vi "Compression with DCT.vi"() -> ()   [LabVIEW 2023]
doc: "This VI uses the DCT VI to compress images. LabVIEW transforms the Source Image to DCT Coefficients in 8-by-8 blocks, then the inverse DCT transforms the image back to Restored Image."
uses:
  Images/_Images.ctl
  <vilib>/Analysis/2dsp.llb/2D DCT.vi
  <vilib>/Analysis/2dsp.llb/2D Inverse DCT.vi
  <vilib>/Analysis/NI_AALPro.lvlib
panel:
  in  "Image Selector":T1=enum."Part1"
  out "DCT":T2(plugin-control)
  in  "Compression Level (1-max, 15 - min)":i32(slide)=4 scale=1.0..15.0
  out "min value":dbl
  out "max value":dbl
  out "Difference":T2(plugin-control)
  out "MSE":dbl
  out "PSNR (dB)":dbl
  out "Reconstructed Image":T2(plugin-control)
  out "Image":T2(plugin-control)
  out "Number of block size":i32
  out "Truncated Pattern":bool[][](array[boolean])=[[TRUE, TRUE, TRUE, TRUE, FALSE, FALSE, FALSE, FALSE], [TRUE, TRUE, TRUE, FALSE, FALSE, FALSE, FALSE, FALSE], [TRUE, TRUE, FALSE, FALSE, FALSE, FALSE, FALSE, FALSE], [TRUE, FALSE, FALSE, FALSE, FALSE, FALSE, FALSE, FALSE], [FALSE, FALSE, FALSE, FALSE, FALSE, FALSE, FALSE, FALSE], [FALSE, FALSE, FALSE, FALSE, FALSE, FALSE, FALSE, FALSE], [FALSE, FALSE, FALSE, FALSE, FALSE, FALSE, FALSE, FALSE], [FALSE, FALSE, FALSE, FALSE, FALSE, FALSE, FALSE, FALSE]]
  # "Image Compression and the Discrete Cosine Transform"
  # "Inverse DCT"
  # "DCT\n(8 X 8 block)"
  # "Modify the Truncated Pattern  and verify \nthat the Mean Square Error (MSE) \nreduces as you enable more bits."
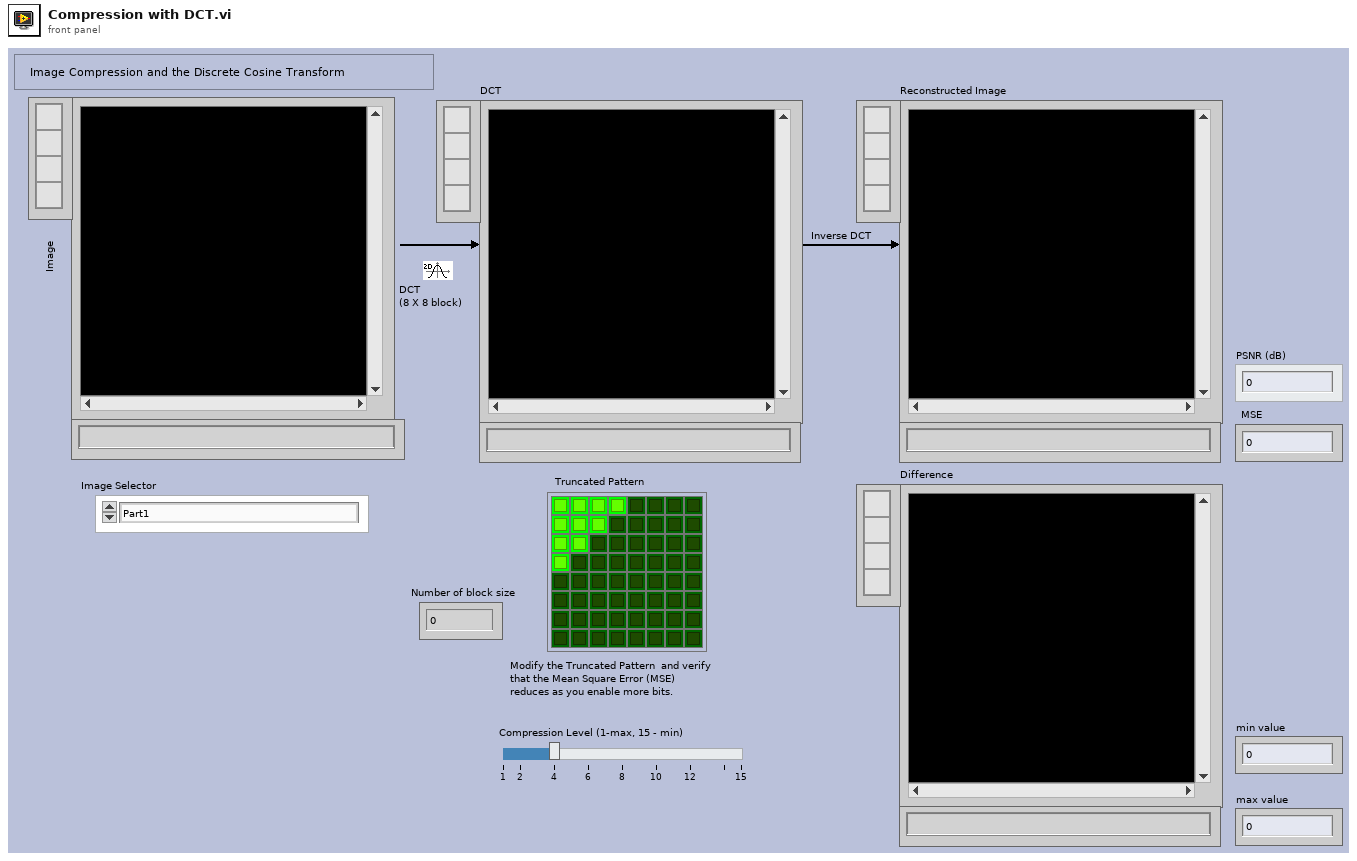
[diagram p1: front panel]
types:
  T1 = typedef "_Images.ctl" = enum16{"Balls2", "Battery1", "Battery2", "Connector1", "Subwoofer1", "Subwoofer2", "Subwoofer3", "Subwoofer4", "Hase1", "Lamp1", "Lamp2", "Mouse1", "PhotoLens1", "Po1", "PowerSupply1", "Router", "--- Step Wedges ---", "Stepwedge1", "Stepwedge2", "Stepwedge3", "--- Fusion ---", "Fusion160kV", "Fusion2-120kV", "Fusion2-320kV", "Fusion300kV", "FusionPart1-120kV", "FusionPart1-180kV", "--- PART 01 ---", "Part1", "Part2", "Part3", "Part4", "Part5", "Part6", "Part7", "Part8", "--- Different Integrations ---", "Step2737-02Int", "Step2737-04Int", "Step2737-08Int", "Step2737-16Int", "Step2737-32Int", "Step2737-64Int"}
  T2 = typedef "IMAQ Image.ctl" = refnum<image>
  T3 = typedef "Image Type" = u32
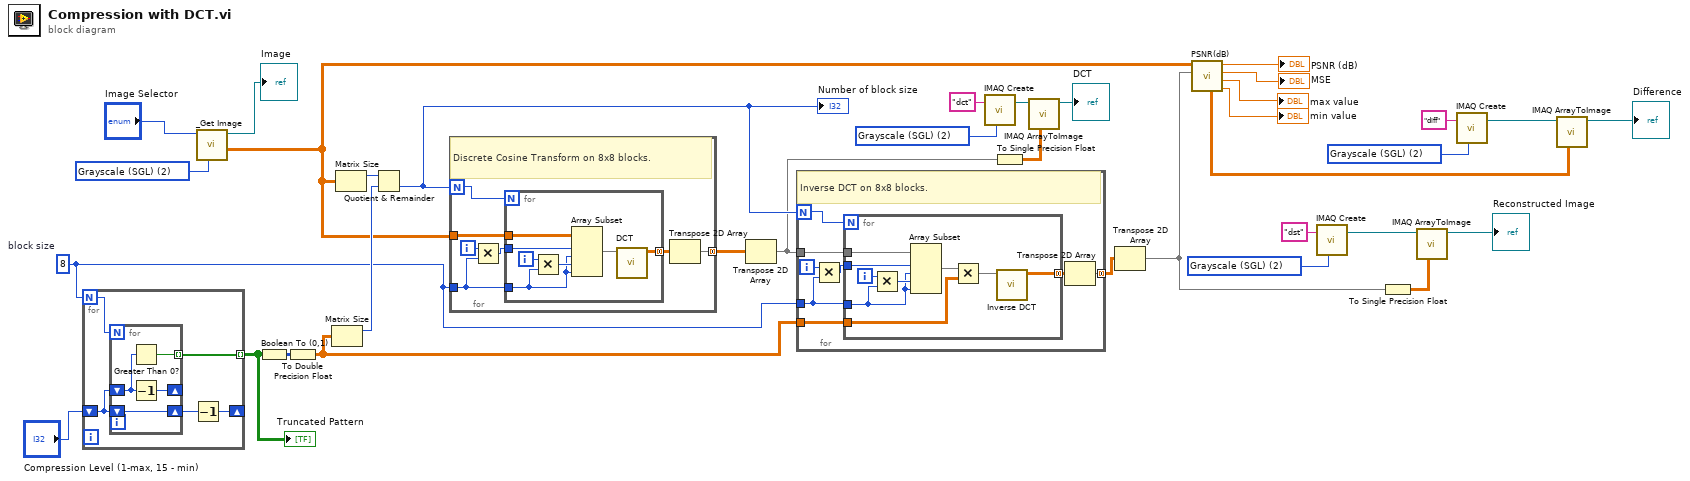
[diagram p0: block diagram]
diagram:
  w11 = T3 2 items=["Grayscale (U8)", "Grayscale (I16)", "Grayscale (SGL)", "Complex (CSG)", "RGB (U32)", "HSL (U32)", "RGB (U64)", "Grayscale (U16)"] ("Image Type")
  w19 = T3 2 items=["Grayscale (U8)", "Grayscale (I16)", "Grayscale (SGL)", "Complex (CSG)", "RGB (U32)", "HSL (U32)", "RGB (U64)", "Grayscale (U16)"] ("Image Type")
  w24 = T3 2 items=["Grayscale (U8)", "Grayscale (I16)", "Grayscale (SGL)", "Complex (CSG)", "RGB (U32)", "HSL (U32)", "RGB (U64)", "Grayscale (U16)"] ("Image Type (U16)")
  w26 = T3 2 items=["Grayscale (U8)", "Grayscale (I16)", "Grayscale (SGL)", "Complex (CSG)", "RGB (U32)", "HSL (U32)", "RGB (U64)", "Grayscale (U16)"] ("Image Type")
  w5 = 8  # block size
  n1 = for {
    N: w5 -> [w40]
    shift-right: [w37] -> _
    shift-left: "Compression Level (1-max, 15 - min)" -> [w38]
    tunnel: [w36] -> w14 mode=indexing
    n2 = for {
      N: w40 -> [_]
      shift-right: [w44] -> w39
      shift-left: w38 -> [w44]
      shift-right: [w43] -> _
      shift-left: w38 -> [w42]
      tunnel: [w41] -> w36 mode=indexing
      n3 = Greater Than 0?(x=w42) -> (x > 0?=w41:bool)
      n4 = Decrement(x=w42) -> (x-1=w43:i32)
    }
    n5 = Decrement(x=w39) -> (x-1=w37:i32)
  }
  "Truncated Pattern" <- w14
  n6 = call "_Get Image.vi"("Image Type (U16)"=w24, "Image"="Image Selector") -> ("Image Pixels (Float)"=w17:dbl[][], "Image Out"=→"Image":T2)  [unwired: 6 in, 2 out]
  n7 = Boolean To (0,1)(Boolean=w14) -> (0, 1=w34:i16[][])
  n8 = To Double Precision Float(number=w34) -> (double precision float=w31:dbl[][])
  n9 = Matrix Size(0:w31) -> (1:w29:i32)  [unwired: 1 out]
  n10 = Matrix Size(0:w17) -> (1:w33:i32)  [unwired: 1 out]
  n11 = Quotient & Remainder(x=w33, y=w29) -> (floor(x/y)=w30:i32)  [unwired: 1 out]
  "Number of block size" <- w30
  n12 = for {
    N: w30 -> [w51]
    tunnel: w17 -> [w50]
    tunnel: [w48] -> w35 mode=concatenating
    tunnel: w5 -> [w46]
    i -> [w47]
    # "Discrete Cosine Transform on 8x8 blocks."
    n13 = Multiply(x=w47, y=w46) -> (x*y=w45:i32)
    n14 = for {
      N: w51 -> [_]
      tunnel: w45 -> [w58]
      tunnel: w50 -> [w57]
      tunnel: [w55] -> w49 mode=concatenating
      tunnel: w46 -> [w52]
      i -> [w53]
      n15 = Multiply(x=w53, y=w52) -> (x*y=w54:i32)
      n16 = Array Subset(array=w57, index (row)=w58, length (row)=w52, index (col)=w54, length (col)=w52) -> (w56:dbl[][])
      n17 = call-poly <vilib>:"DCT.vi"("X"=w56) -> ("DCT {X}"=w55:dbl[][])  [unwired: 9 in, 1 out]
    }
    n18 = Transpose 2D Array(2D array=w49) -> (transposed array=w48:dbl[][])
  }
  n19 = Transpose 2D Array(2D array=w35) -> (transposed array=w9:dbl[][])
  n20 = for {
    N: w30 -> [w66]
    tunnel: w9 -> [w65]
    tunnel: [w63] -> w32 mode=concatenating
    tunnel: w5 -> [w61]
    tunnel: w31 -> [w59]
    i -> [w62]
    # "Inverse DCT on 8x8 blocks."
    n21 = Multiply(x=w62, y=w61) -> (x*y=w60:i32)
    n22 = for {
      N: w66 -> [_]
      tunnel: w60 -> [w75]
      tunnel: w65 -> [w74]
      tunnel: [w67] -> w64 mode=concatenating
      tunnel: w61 -> [w71]
      tunnel: w59 -> [w69]
      i -> [w72]
      n23 = Multiply(x=w72, y=w71) -> (x*y=w73:i32)
      n24 = Array Subset(array=w74, index (row)=w75, length (row)=w71, index (col)=w73, length (col)=w71) -> (w68:dbl[][])
      n25 = Multiply ("Multiply.vi")(x=w68, y=w69) -> (x*y=w70:dbl[][])
      n26 = call-poly <vilib>:"Inverse DCT.vi"("DCT {X}"=w70) -> ("X"=w67:dbl[][])  [unwired: 9 in, 1 out]
    }
    n27 = Transpose 2D Array(2D array=w64) -> (transposed array=w63:dbl[][])
  }
  n28 = call "IMAQ Create"("Image Name"="dct", "Image Type"=w11) -> ("New Image"=w12:T2)  [unwired: 3 in, 1 out]
  n29 = To Single Precision Float(number=w9) -> (single precision float=w13:sgl[][])
  n30 = call "IMAQ ArrayToImage"("Image Pixels (Float)"=w13, "Image"=w12) -> ("Image Out"=→"DCT":T2)  [unwired: 8 in, 1 out]
  n31 = Transpose 2D Array(2D array=w32) -> (transposed array=w16:dbl[][])
  n32 = call "PSNR(dB).vi"("Image Pixels (Float) 2"=w16, "Image Pixels (Float) 1"=w17) -> ("min diff"=→"min value":dbl, "max diff"=→"max value":dbl, "Mean Square Error (MSE)"=→"MSE":dbl, "PSNR (dB)"=→"PSNR (dB)":dbl, "Difference"=w8:sgl[][])  [unwired: 5 in]
  n33 = call "IMAQ Create"("Image Name"="dst", "Image Type"=w26) -> ("New Image"=w25:T2)  [unwired: 3 in, 1 out]
  n34 = To Single Precision Float(number=w16) -> (single precision float=w23:sgl[][])
  n35 = call "IMAQ ArrayToImage"("Image Pixels (Float)"=w23, "Image"=w25) -> ("Image Out"=→"Reconstructed Image":T2)  [unwired: 8 in, 1 out]
  n36 = call "IMAQ Create"("Image Name"="diff", "Image Type"=w19) -> ("New Image"=w20:T2)  [unwired: 3 in, 1 out]
  n37 = call "IMAQ ArrayToImage"("Image Pixels (Float)"=w8, "Image"=w20) -> ("Image Out"=→"Difference":T2)  [unwired: 8 in, 1 out]
